vi "Dart Auto V.3.0.vi"() -> (3 "Stop":bool=TRUE)   [LabVIEW 2017]
uses:
  Robot Global Data V.3.0.vi
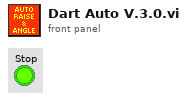
[diagram p1: front panel]
types:
  T1 = cluster{"Pot. Voltage":dbl[], "Corresponding Inches":dbl[]}
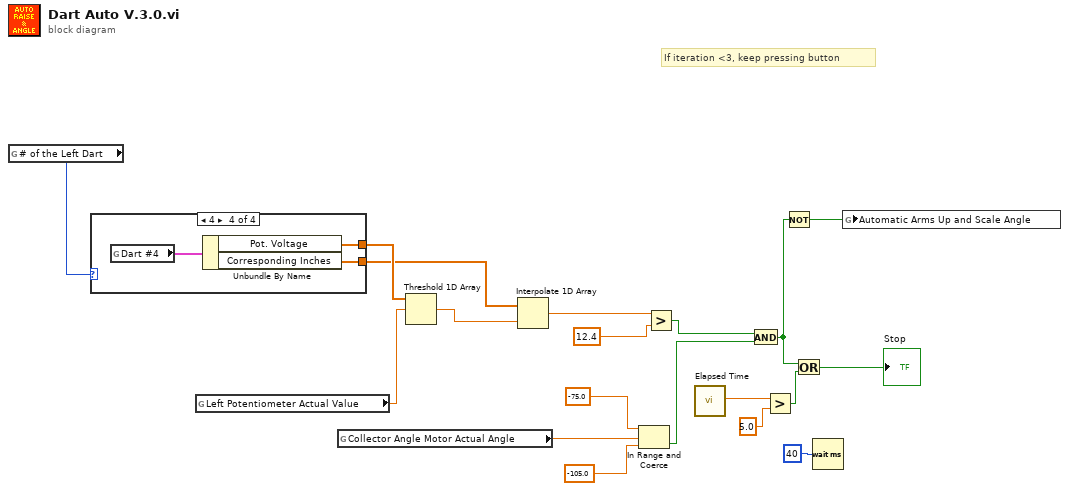
[diagram p0: block diagram]
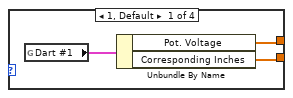
[diagram p2: hidden frame]
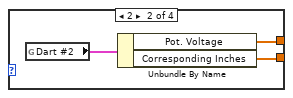
[diagram p3: hidden frame]
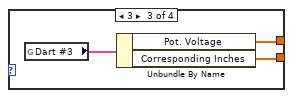
[diagram p4: hidden frame]
diagram:
  # "If iteration <3, keep pressing button"
  n1 = global read "Robot Global Data V.3.0.vi" "# of the Left Dart"() -> (w8:i32)
  n2 = case shown="4" w8 {
    tunnel: [w21 w24 w27 w30] -> w10
    tunnel: [w20 w23 w26 w29] -> w9
    frame 1, Default {
      n3 = global read "Robot Global Data V.3.0.vi" "Dart #1"() -> (w22:T1)
      n4 = Unbundle By Name(w22) -> ("Pot. Voltage"=w21:dbl[], "Corresponding Inches"=w20:dbl[])
    }
    frame 2 {
      n5 = global read "Robot Global Data V.3.0.vi" "Dart #2"() -> (w25:T1)
      n6 = Unbundle By Name(w25) -> ("Pot. Voltage"=w24:dbl[], "Corresponding Inches"=w23:dbl[])
    }
    frame 3 {
      n7 = global read "Robot Global Data V.3.0.vi" "Dart #3"() -> (w28:T1)
      n8 = Unbundle By Name(w28) -> ("Pot. Voltage"=w27:dbl[], "Corresponding Inches"=w26:dbl[])
    }
    frame 4 {
      n9 = global read "Robot Global Data V.3.0.vi" "Dart #4"() -> (w31:T1)
      n10 = Unbundle By Name(w31) -> ("Pot. Voltage"=w30:dbl[], "Corresponding Inches"=w29:dbl[])
    }
  }
  n11 = global read "Robot Global Data V.3.0.vi" "Left Potentiometer Actual Value"() -> (w11:dbl)
  n12 = global read "Robot Global Data V.3.0.vi" "Collector Angle Motor Actual Angle"() -> (w17:dbl)
  n13 = Threshold 1D Array(2:w11, 3:w10) -> (0:w12:dbl)  [unwired: 1 in]
  n14 = Interpolate 1D Array(1:w12, 2:w9) -> (0:w7:dbl)
  n15 = In Range and Coerce(upper limit=-75.0, x=w17, lower limit=-105.0) -> (In Range?=w14:bool)  [unwired: 1 out]
  n16 = Greater?(x=w7, y=12.4) -> (0:w18:bool)
  n17 = call "Elapsed Time"() -> ("Elapsed Time (s)"=w4:dbl)  [unwired: 12 in, 7 out]
  n18 = And(x=w18, y=w14) -> (x .and. y?=w2:bool)
  n19 = Greater?(x=w4, y=5.0) -> (0:w3:bool)
  n20 = Not(x=w2) -> (.not. x?=w6:bool)
  n21 = Or(x=w2, y=w3) -> (x .or. y?=→"Stop":bool)
  n22 = Wait (ms)(milliseconds to wait=u32 40) -> ()  [unwired: 1 out]
  n23 = global write "Robot Global Data V.3.0.vi" "Automatic Arms Up and Scale Angle"(w6) -> ()
